vi "e.gate HighSpeedPort Error Handler.vi"(6 "error code start index":i32, 7 "VI reference":refnum<vi>, 8 "error in (no error)":errorcluster, 11 "binary data in":u8[](array[numeric])) -> (0 "error out":errorcluster, 3 "binary out":u8[](array[numeric]))   [LabVIEW 2016]
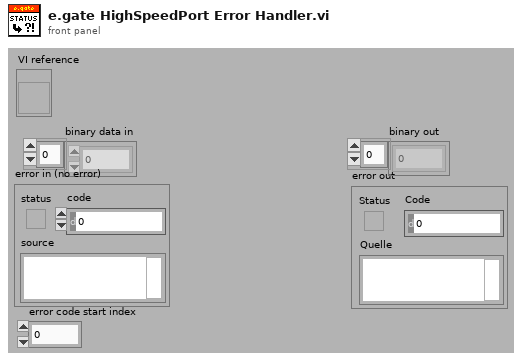
[diagram p1: front panel]
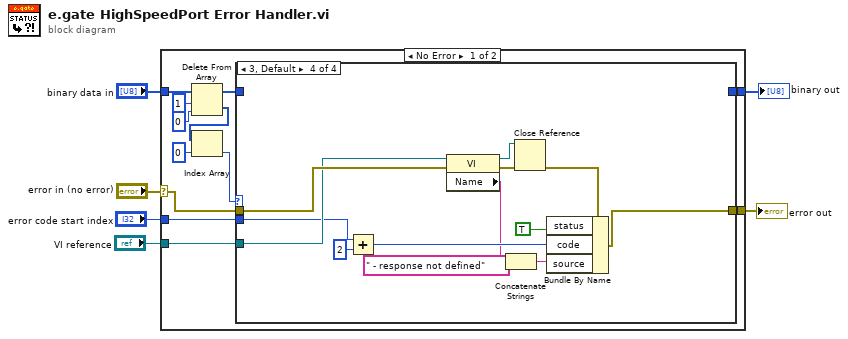
[diagram p0: block diagram]
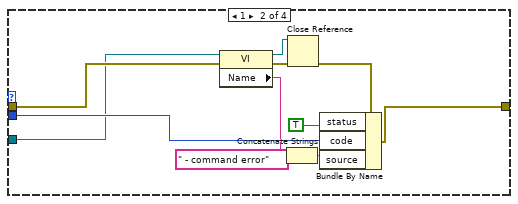
[diagram p3: hidden frame]
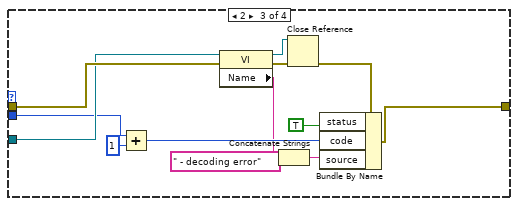
[diagram p4: hidden frame]
diagram:
  n1 = case shown="No Error" "error in (no error)" {
    selector: "error in (no error)" -> [w12 w58]
    tunnel: "binary data in" -> [w14 _]
    tunnel: "error code start index" -> [w11 _]
    tunnel: [w10 w58] -> w3
    tunnel: [w8 _] -> w2
    tunnel: "VI reference" -> [w7 _]
    frame No Error {
      n2 = Delete From Array(array=w14, length=1 ("Länge"), index=0 ("Index")) -> (deleted portion=w15:u8[], array with subset deleted=w9:u8[])
      n3 = Index Array(array=w15, index=0 ("Index")) -> (element=w13:u8)
      n4 = case shown="3, Default" w13 {
        tunnel: w12 -> [w20 w26 w40 w53]
        tunnel: w11 -> [_ w30 w36 w49]
        tunnel: [w20 w29 w43 w56] -> w10
        tunnel: w9 -> [w19 _ _ _]
        tunnel: [w19 _ _ _] -> w8
        tunnel: w7 -> [_ w25 w39 w52]
        frame 0 {
        }
        frame 1 {
          n5 = property class="VI"(reference=w25, error in=w26) -> (reference out=w27:refnum<vi>, error out=w28:errorcluster, "Name"=w22:string)
          n6 = Concatenate Strings(w22, " - command error" ("String")) -> (w23:string)
          n7 = Close Reference(reference=w27, error in (no error)=w28) -> (error out=w24:errorcluster)
          n8 = Bundle By Name(cluster=w24, "status"=TRUE, "code"=w30, "source"=w23) -> (w29:errorcluster)
        }
        frame 2 {
          n9 = Add(x=w36, y=1) -> (x+y=w35:i32)
          n10 = property class="VI"(reference=w39, error in=w40) -> (reference out=w41:refnum<vi>, error out=w42:errorcluster, "Name"=w33:string)
          n11 = Concatenate Strings(w33, " - decoding error" ("String")) -> (w34:string)
          n12 = Close Reference(reference=w41, error in (no error)=w42) -> (error out=w38:errorcluster)
          n13 = Bundle By Name(cluster=w38, "status"=TRUE, "code"=w35, "source"=w34) -> (w43:errorcluster)
        }
        frame 3, Default {
          n14 = Add(x=w49, y=2) -> (x+y=w48:i32)
          n15 = property class="VI"(reference=w52, error in=w53) -> (reference out=w54:refnum<vi>, error out=w55:errorcluster, "Name"=w46:string)
          n16 = Concatenate Strings(w46, " - response not defined" ("String")) -> (w47:string)
          n17 = Close Reference(reference=w54, error in (no error)=w55) -> (error out=w51:errorcluster)
          n18 = Bundle By Name(cluster=w51, "status"=TRUE, "code"=w48, "source"=w47) -> (w56:errorcluster)
        }
      }
    }
    frame Error {
    }
  }
  "error out" <- w3
  "binary out" <- w2
